vi "Global_CMD Data.vi"() -> ()   [LabVIEW 2017, in "VisionSystem.lvlib"]
uses:
  VisionSystem.lvlib
  Cluster_CMD to Vision.ctl
  Enum_ Field Targets.ctl
panel:
  in  "CMD_Camera Data":T1
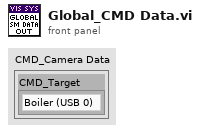
[diagram p1: front panel]
types:
  T1 = typedef "VisionSystem.lvlib/Cluster_CMD to Vision.ctl" = cluster{"CMD_Target":T2}
  T2 = typedef "VisionSystem.lvlib/Enum_ Field Targets.ctl" = enum16{"Boiler (USB 0)", "Rope (USB 1)"}
diagram:
